vi "initialize.vi"(8 "error in (no error)":errorcluster, 11 "Experiment in":refnum<class "Experiment.lvclass">) -> (0 "error out":errorcluster, 3 "Experiment out":refnum<class "Experiment.lvclass">)   [LabVIEW 2013, in "Experiment.lvclass"]
uses:
  Experiment.lvclass
  Experiment.lvclass/Experiment.ctl
  Camera/Hamamatsu_C9100-13/Hamamatsu_C9100-13.lvclass
  Globals.vi
  HSDIO/HSDIO.lvclass
  Counter/Counter.lvclass
  PI_piezo/PI_Piezo.lvclass
  TTL_input/TTL_input.lvclass
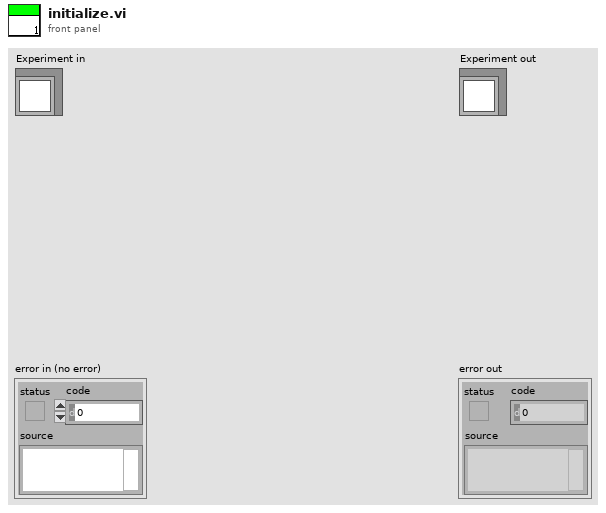
[diagram p1: front panel]
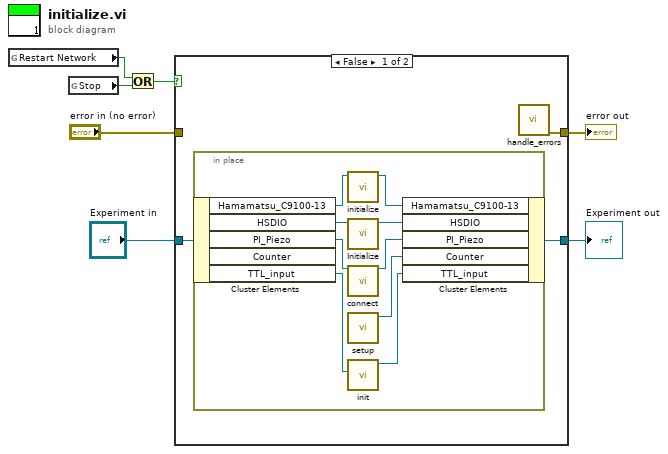
[diagram p0: block diagram]
diagram:
  n1 = global read "Globals.vi" "Restart Network"() -> (w4:bool)
  n2 = global read "Globals.vi" "Stop"() -> (w3:bool)
  n3 = Or(x=w4, y=w3) -> (x .or. y?=w2:bool)
  n4 = case shown="False" w2 {
    tunnel: [w8 w20] -> w7
    tunnel: [w9 w21] -> w5
    tunnel: "Experiment in" -> [w10 w21]
    tunnel: "error in (no error)" -> [_ w20]
    frame False {
      n5 = in-place {
        n6 = in-place-cluster #1(w10) -> ("Hamamatsu_C9100-13"=w19:refnum<class "Hamamatsu_C9100-13.lvclass">, "HSDIO"=w16:refnum<class "HSDIO.lvclass">, "PI_Piezo"=w15:refnum<class "PI_Piezo.lvclass">, "TTL_input"=w11:refnum<class "TTL_input.lvclass">)  [unwired: 1 out]
        n7 = call-dynamic "initialize.vi"("Hamamatsu_C9100-13 in"=w19) -> ("Hamamatsu_C9100-13 out"=w18:refnum<class "Hamamatsu_C9100-13.lvclass">)  [unwired: 9 in, 1 out]
        n8 = call "Initialize.vi"("HSDIO in"=w16) -> ("HSDIO out"=w17:refnum<class "HSDIO.lvclass">)  [unwired: 9 in, 1 out]
        n9 = call "connect.vi"("PI_Piezo.lvclass (in)"=w15) -> ("PI_Piezo.lvclass"=w14:refnum<class "PI_Piezo.lvclass">)  [unwired: 13 in, 1 out]
        n10 = call "setup.vi"() -> ("Counter out"=w13:refnum<class "Counter.lvclass">)  [unwired: 10 in, 1 out]
        n11 = call "init.vi"("TTL_input.lvclass"=w11) -> ("TTL_input out"=w12:refnum<class "TTL_input.lvclass">)  [unwired: 9 in, 1 out]
        n12 = in-place-cluster #1("Hamamatsu_C9100-13"=w18, "HSDIO"=w17, "PI_Piezo"=w14, "Counter"=w13, "TTL_input"=w12) -> (w9:refnum<class "Experiment.lvclass">)
      }
      n13 = call "handle_errors.vi"() -> ("error out"=w8:errorcluster)  [unwired: 15 in]
    }
    frame True {
    }
  }
  "error out" <- w7
  "Experiment out" <- w5
